vi "ctx set correlation fifo temp directory.vi"(11 "directory":string) -> (3 "function return":i32)   [LabVIEW 2019, in "apdm.lvlib"]
doc: "APDM_EXPORT int apdm_ctx_set_correlation_fifo_temp_directory(const char *directory);"
uses:
  apdm.lvlib
  Lee Lab/CP FES Walking 2018/Code/Working/LabVIEW/apdm.dll
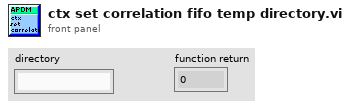
[diagram p1: front panel]
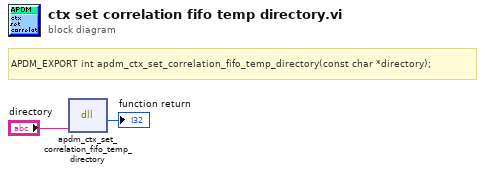
[diagram p0: block diagram]
diagram:
  # "APDM_EXPORT int apdm_ctx_set_correlation_fifo_temp_directory(const char *directory);"
  n1 = dll-call lib="C:/Users/jfalesi/Dropbox/Lee Lab/CP FES Walking 2018/Code/Working/LabVIEW/apdm.*" fn="apdm_ctx_set_correlation_fifo_temp_directory"("directory"="directory") -> (→"function return":i32)  [unwired: 4 in, 2 out]
